vi "Get SMO Port.vi"(8 "error in (no error)":errorcluster, 11 "Instrument.AFM_DLog in":refnum<class "Instrument.AFM_DLog.lvclass">) -> (0 "error out":errorcluster, 2 "Port":u16, 3 "Instrument.AFM_DLog out":refnum<class "Instrument.AFM_DLog.lvclass">)   [LabVIEW 2019, in "Instrument.AFM_DLog.lvclass"]
uses:
  Instrument.AFM_DLog.lvclass
  <userlib>/LevyLab/Instrument Framework/Instrument Types/SCPI/Instrument.SCPI.lvclass
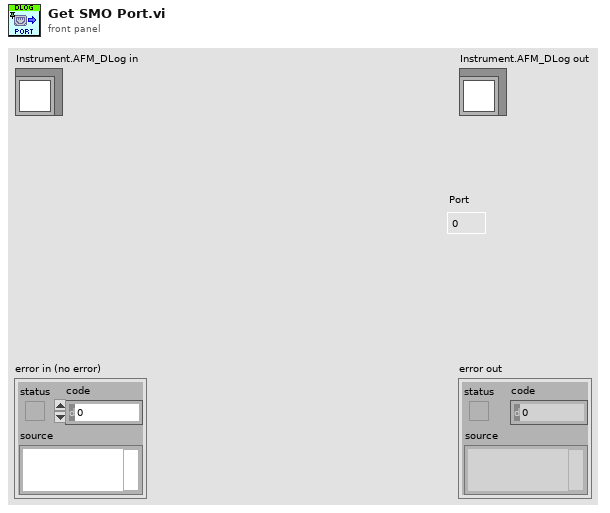
[diagram p1: front panel]
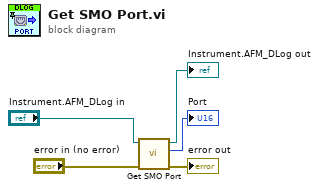
[diagram p0: block diagram]
diagram:
  n1 = call-parent "Get SMO Port.vi"("error in (no error)"="error in (no error)", "Instrument in"="Instrument.AFM_DLog in") -> ("error out"=→"error out":errorcluster, "Port"=→"Port":u16, "Instrument out"=→"Instrument.AFM_DLog out":refnum<class "Instrument.AFM_DLog.lvclass">)  [unwired: 7 in]
